vi "Start Async Call Template.vi"   [LabVIEW 2017]
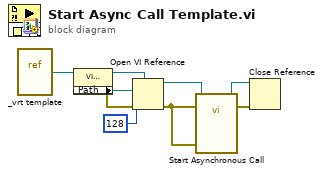
[diagram p0: block diagram]
diagram:
  n1 = vi-ref "_vrt template.vi"() -> (w7:refnum<vi>)
  n2 = property class="VI (strict)"(reference=w7) -> (reference out=w3:refnum<vi>, error out=w5:errorcluster, "Path"=w6:path)  [unwired: 1 in]
  n3 = Open VI Reference(type specifier VI Refnum (for type only)=w3, vi path=w6, options=128, error in (no error)=w5) -> (vi reference=w8:refnum<vi>, error out=w2:errorcluster)  [unwired: 2 in]
  n4 = call-by-ref "Start Asynchronous Call"(reference=w8, error in=w2, 8:"error in (no error)"=w2) -> (reference out=w9:refnum<vi>, error out=w4:errorcluster)  [unwired: 10 in, 1 out]
  n5 = Close Reference(reference=w9, error in (no error)=w4) -> ()  [unwired: 1 out]
